vi "ManipWaitForAlignment.vi"(2 "Reinit":bool) -> (0 "error out":errorcluster, 1 "Advance Trigger":bool)   [LabVIEW 2020]
doc: "This VI requires the maniplator sequencer to wait until the arm has reached its goal position.\n\nParameters:\nNone"
uses:
  SafeParser_Integer.vi
  GlobalPoseAndTargeting.vi
panel:
  in  "Parameter String":string
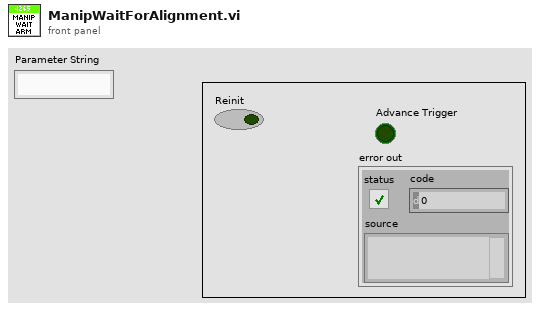
[diagram p1: front panel]
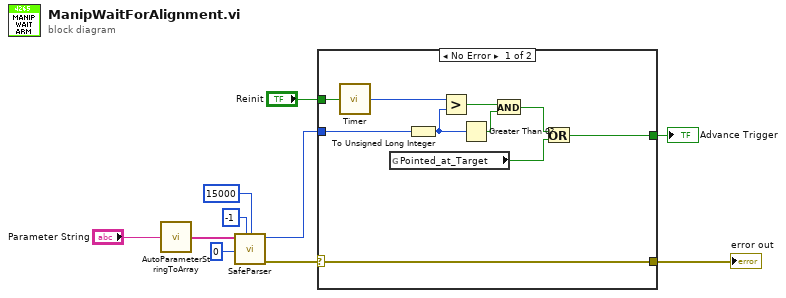
[diagram p0: block diagram]
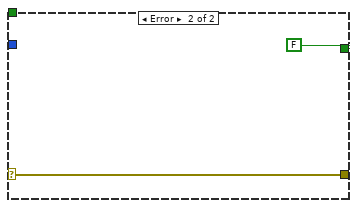
[diagram p2: hidden frame]
diagram:
  n1 = call "AutoParameterStringToArray.vi"("Parameter String"="Parameter String") -> ("Parsed Parameters"=w3:string[])
  n2 = call-poly "SafeParser.vi"("Maximum"=15000, "Minimum"=-1, "Array Index"=0 ("Parameter Index"), "String Array"=w3) -> ("Error Out"=w2:errorcluster, "Typecast  Value"=w1:i32)  [unwired: 6 in]
  n3 = case shown="No Error" w2 {
    selector: w2 -> [w20 w21]
    tunnel: [w11 FALSE] -> w10
    tunnel: [w20 w21] -> w9
    tunnel: w1 -> [w15 _]
    tunnel: "Reinit" -> [w14 _]
    frame No Error {
      n4 = call "Timer.vi"("Reset Timer"=w14) -> ("Time (ms)"=w16:u32)
      n5 = global read "GlobalPoseAndTargeting.vi" "Pointed_at_Target"() -> (w12:bool)
      n6 = To Unsigned Long Integer(number=w15) -> (unsigned 32bit integer=w17:u32)
      n7 = Greater?(x=w16, y=w17) -> (0:w19:bool)
      n8 = Greater Than 0?(x=w17) -> (x > 0?=w18:bool)
      n9 = And(x=w19, y=w18) -> (x .and. y?=w13:bool)
      n10 = Or(x=w13, y=w12) -> (x .or. y?=w11:bool)
    }
    frame Error {
    }
  }
  "Advance Trigger" <- w10
  "error out" <- w9
